vi "Chart-Set Overview Limit.vi"(8 "error in":errorcluster, 10 "Limit":cluster{"Lower Limit":dbl, "Upper Limit":dbl}, 11 "Overview Refnum In":refnum<vi>) -> (0 "error out":errorcluster, 3 "Overview Refnum Out":refnum<vi>)   [LabVIEW 2020]
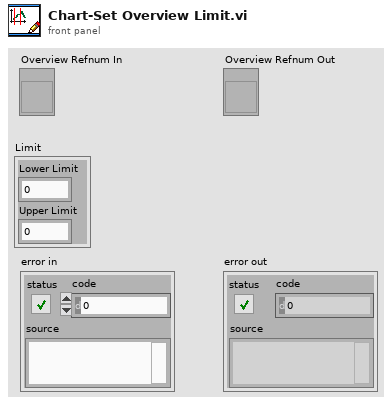
[diagram p1: front panel]
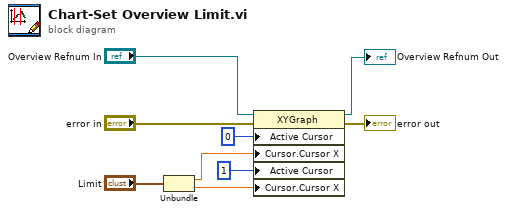
[diagram p0: block diagram]
diagram:
  n1 = Unbundle("Limit") -> ("Lower Limit"=w4:dbl, "Upper Limit"=w3:dbl)
  n2 = property class="XYGraph"(reference="Overview Refnum In", error in="error in", "Active Cursor"=u32 0, "Cursor.Cursor X"=w4, "Active Cursor"=u32 1, "Cursor.Cursor X"=w3) -> (reference out=→"Overview Refnum Out":refnum<vi>, error out=→"error out":errorcluster)
